vi "Time_Trak.vi"() -> ()   [LabVIEW 2013]
uses:
  Support/LV_File.lvclass
  Support/File.lvclass
panel:
  out "Modules":T1(array[cluster])
  in  "Pause":bool
  in  "New Module":bool
  in  "Stop":bool
  in  "Start":bool
  # "this code still has a lot of bugs to work out, but there is some promising aspects as well"
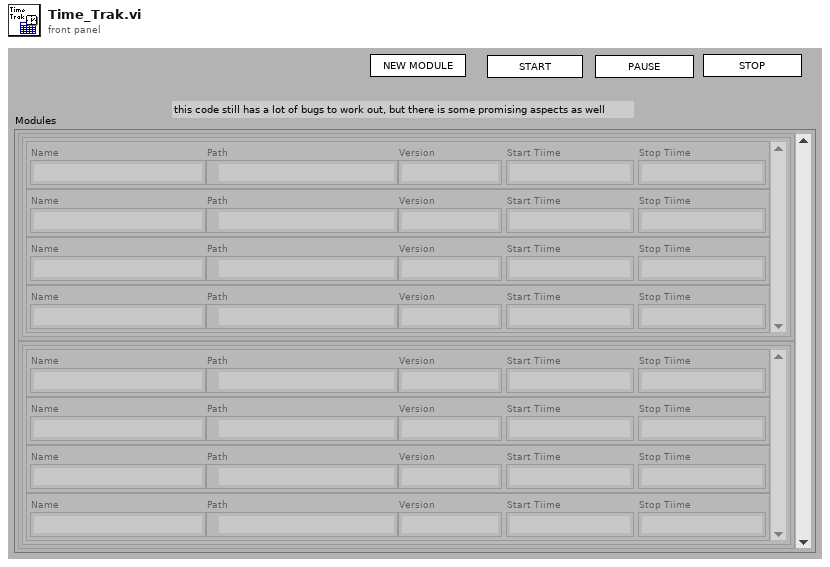
[diagram p1: front panel]
types:
  T1 = cluster{"Module":cluster{"Name":string, "Path":path, "Version":string, "Start Tiime":string, "Stop Tiime":string}[]}[]
  T2 = cluster{"Name":string, "Path":path, "Version":string, "Start Tiime":string, "Stop Tiime":string}
  T3 = cluster{"Module":cluster{"Name":string, "Path":path, "Version":string, "Start Tiime":string, "Stop Tiime":string}[]}
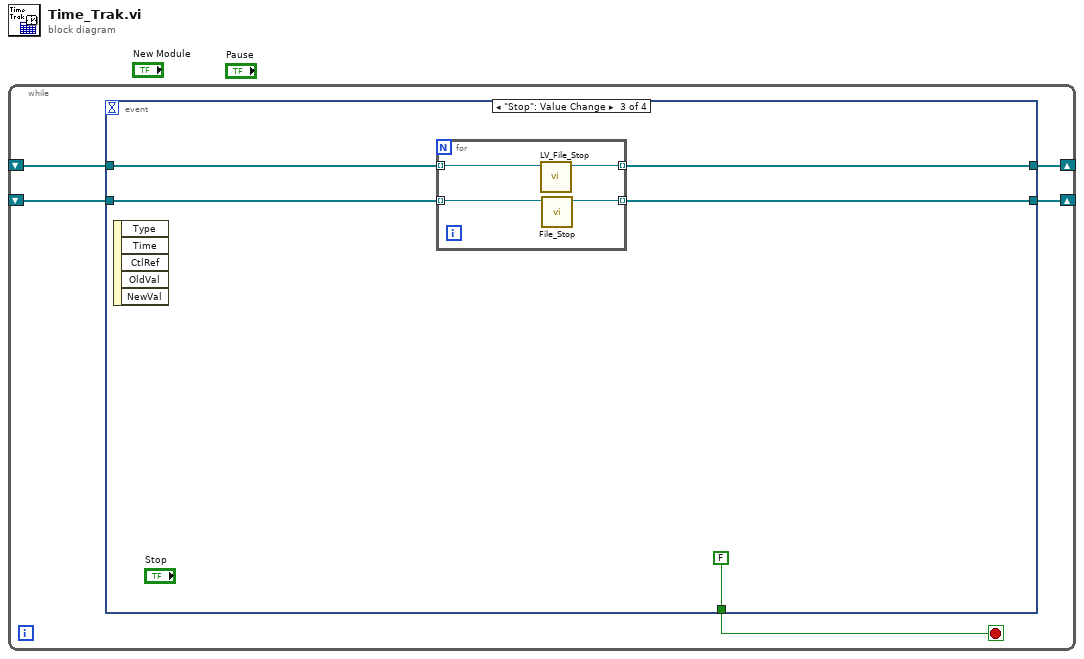
[diagram p0: block diagram]
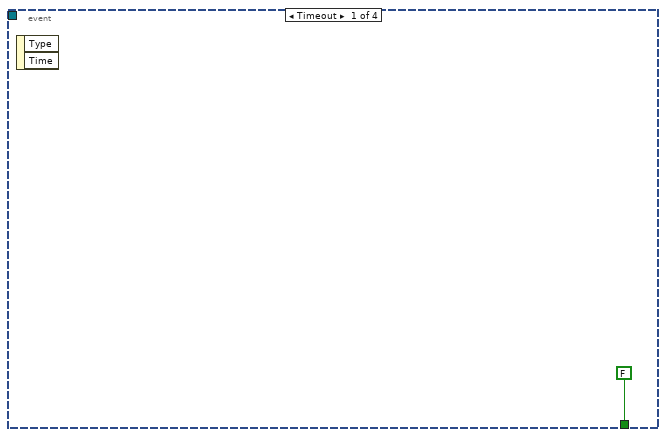
[diagram p2: hidden frame]
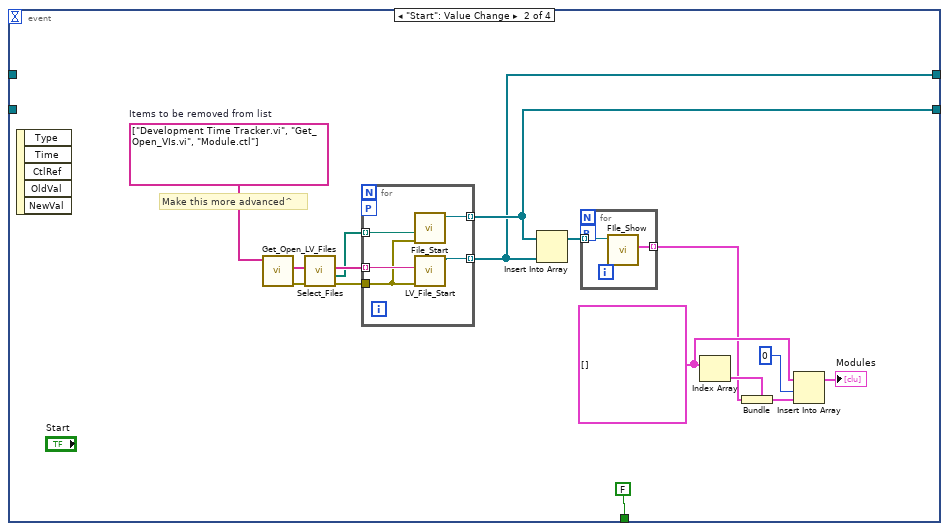
[diagram p3: hidden frame]
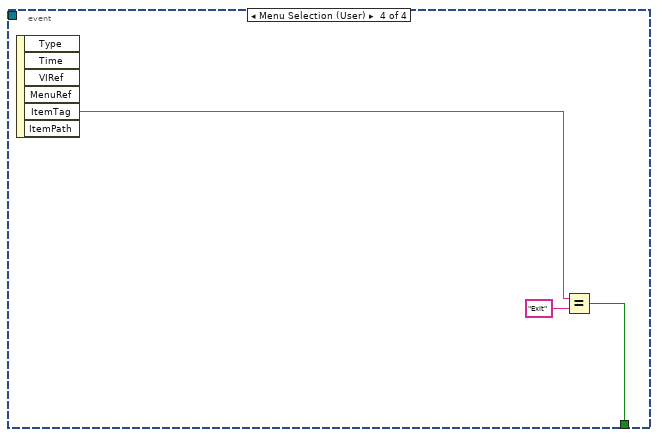
[diagram p4: hidden frame]
diagram:
  n1 = while {
    shift-right: [w4] -> _
    shift-left: _ -> [w3]
    shift-right: [w2] -> _
    shift-left: _ -> [w1]
    stop <- w5 stop-if-true
    n2 = event shown="[2] \"Stop\": Value Change" {
      selector: _ -> [_ _ _ _]
      dyn-events: _ -> [_ _ _ _]
      timeout: _ -> [_ _ _ _]
      tunnel: [FALSE FALSE FALSE w41] -> w5
      tunnel: [_ w14 w31 _] -> w4
      tunnel: w3 -> [_ _ w32 _]
      tunnel: [_ w13 w30 _] -> w2
      tunnel: w1 -> [_ _ w33 _]
      event Timeout {
        n3 = event-data() -> ()  [unwired: 1 in, 2 out]
      }
      event "Start": Value Change {
        w10 = T1 [] ("Modules")
        w17 = string[] ["Development Time Tracker.vi", "Get_Open_VIs.vi", "Module.ctl"]  # Items to be removed from list
        # "Make this more advanced^"
        n4 = event-data() -> ()  [unwired: 1 in, 5 out]
        n5 = call "Get_Open_LV_Files.vi"("Items to be ignored"=w17) -> ("error out"=w19:errorcluster, "Application:All VIs In Memory"=w18:string[])  [unwired: 9 in]
        n6 = call "Select_Files.vi"("error in"=w19, "Select Files"=w18) -> ("error out"=w15:errorcluster, "Selected External File Paths"=w16:path[], "Selected LV Files"=w20:string[])  [unwired: 7 in]
        n7 = for {
          tunnel: w20 -> [w29] mode=indexing
          tunnel: [w28] -> w13 mode=indexing
          tunnel: w16 -> [w27] mode=indexing
          tunnel: [w26] -> w14 mode=indexing
          tunnel: w15 -> [w25]
          workers-P: _ -> [_]
          n8 = call "File_Start.vi"("error in"=w25, "Path"=w27) -> ("File.lvclass (OUT)"=w26:refnum<class "File.lvclass">)  [unwired: 8 in, 1 out]
          n9 = call "LV_File_Start.vi"("error in"=w25, "VI Name"=w29) -> ("LV_File.lvclass (OUT)"=w28:refnum<class "LV_File.lvclass">)  [unwired: 8 in, 1 out]
        }
        n10 = Insert Into Array(array=w14, new element=w13) -> (w21:refnum<class "File.lvclass">[])  [unwired: 1 in]
        n11 = for {
          tunnel: [w24] -> w8 mode=indexing
          tunnel: w21 -> [w23] mode=indexing
          workers-P: _ -> [_]
          n12 = call "FIle_Show.vi"("File.lvclass (IN)"=w23) -> ("File"=w24:T2)  [unwired: 8 in, 2 out]
        }
        n13 = Index Array(array=w10) -> (element=w9:T3)  [unwired: 1 in]
        n14 = Bundle(cluster=w9, "Module"=w8) -> (w7:T3)
        n15 = Insert Into Array(array=w10, index=0, new element=w7) -> (→"Modules":T1)
      }
      event "Stop": Value Change {
        n16 = event-data() -> ()  [unwired: 1 in, 5 out]
        n17 = for {
          tunnel: w33 -> [w38] mode=indexing
          tunnel: w32 -> [w37] mode=indexing
          tunnel: [w36] -> w31 mode=indexing
          tunnel: [w35] -> w30 mode=indexing
          n18 = call "LV_File_Stop.vi"("LV_File.lvclass (IN)"=w38) -> ("LV_File.lvclass (OUT)"=w35:refnum<class "LV_File.lvclass">)  [unwired: 9 in, 1 out]
          n19 = call "File_Stop.vi"("File.lvclass (IN)"=w37) -> ("File.lvclass (OUT)"=w36:refnum<class "File.lvclass">)  [unwired: 9 in, 1 out]
        }
      }
      event Menu Selection (User) {
        n20 = event-data() -> ("ItemTag"=w40:string)  [unwired: 1 in, 5 out]
        n21 = Equal?(x=w40, y="Exit") -> (x = y?=w41:bool)
      }
    }
  }
